vi "Andor_iXon_Init_Picture.vi"(8 "Input Cluster 2":T6) -> (0 "Output Cluster":T6)   [LabVIEW 2009]
uses:
  atmcd32d.llb/AcquisitionMode_mode typedef.ctl
  atmcd32d.llb/ReadMode_mode typedef.ctl
  atmcd32d.llb/TriggerMode_mode typedef.ctl
  atmcd32d.llb/Shutter_type typedef.ctl
  atmcd32d.llb/Shutter_mode typedef.ctl
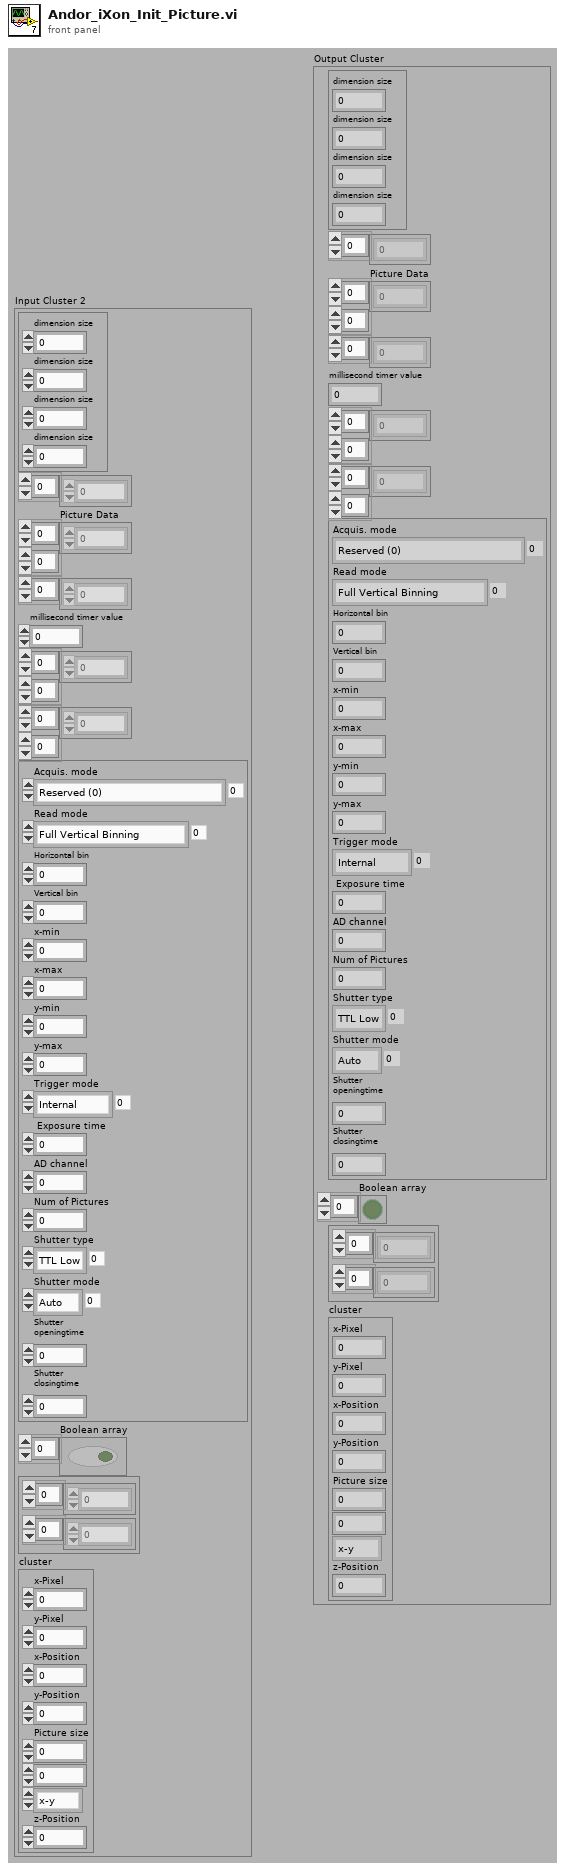
[diagram p1: front panel]
types:
  T1 = typedef "AcquisitionMode_mode typedef.ctl" = enum16{"Reserved (0)", "Single Scan", "Accumulate", "Kinetics", "Fast Kinetics", "Run Till Abort", "Reserved (6)", "Reserved (7)", "Reserved (8)", "Time Delayed Integration"}
  T2 = typedef "ReadMode_mode typedef.ctl" = enum16{"Full Vertical Binning", "Multi-Track", "Random-Track", "Single-Track", "Image"}
  T3 = typedef "TriggerMode_mode typedef.ctl" = enum16{"Internal", "External", "N/A (2)", "N/A (3)", "N/A (4)", "N/A (5)", "External Start"}
  T4 = typedef "Shutter_type typedef.ctl" = enum16{"TTL Low", "TTL High"}
  T5 = typedef "Shutter_mode typedef.ctl" = enum16{"Auto", "Open", "Close"}
  T6 = cluster{cluster{"dimension size":i32, "dimension size":i32, "dimension size":i32, "dimension size":i32}, i32[], "Picture Data":dbl[][], u32[], "millisecond timer value":u32, dbl[][], i32[][], cluster{"Acquis. mode":T1, "Read mode":T2, "Horizontal bin":i32, "Vertical bin":i32, "x-min":i32, "x-max":i32, "y-min":i32, "y-max":i32, "Trigger mode":T3, " Exposure time":sgl, "AD channel":i32, "Num of Pictures":i32, "Shutter type":T4, "Shutter mode":T5, "Shutter\nopeningtime":i32, "Shutter\nclosingtime":i32}, "Boolean array":bool[], cluster{dbl[], dbl[]}, "cluster":cluster{"x-Pixel":u16, "y-Pixel":u16, "x-Position":dbl, "y-Position":dbl, "Picture size":dbl, dbl, enum32{"x-y", "x-z", "y-z"}, "z-Position":dbl}}
  T7 = cluster{"Acquis. mode":T1, "Read mode":T2, "Horizontal bin":i32, "Vertical bin":i32, "x-min":i32, "x-max":i32, "y-min":i32, "y-max":i32, "Trigger mode":T3, " Exposure time":sgl, "AD channel":i32, "Num of Pictures":i32, "Shutter type":T4, "Shutter mode":T5, "Shutter\nopeningtime":i32, "Shutter\nclosingtime":i32}
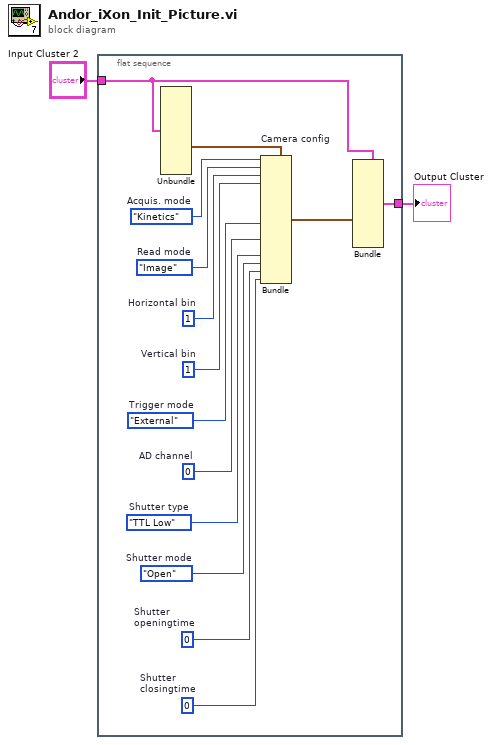
[diagram p0: block diagram]
diagram:
  n1 = flat-sequence {
    tunnel: "Input Cluster 2" -> [w4]
    tunnel: [w6] -> w2
    frame #0 {
      w10 = 1  # Vertical bin
      w9 = 1  # Horizontal bin
      w16 = 0  # Shutter closingtime
      w15 = 0  # Shutter openingtime
      w14 = Shutter_mode_typedef."Open"  # Shutter mode
      w13 = Shutter_type_typedef."TTL Low"  # Shutter type
      w12 = 0  # AD channel
      w11 = TriggerMode_mode_typedef."External"  # Trigger mode
      w8 = ReadMode_mode_typedef."Image"  # Read mode
      w7 = AcquisitionMode_mode_typedef."Kinetics"  # Acquis. mode
      n2 = Unbundle(w4) -> (w3:T7)  [unwired: 10 out]
      n3 = Bundle "Camera config"(cluster=w3, "Acquis. mode"=w7, "Read mode"=w8, "Horizontal bin"=w9, "Vertical bin"=w10, "Trigger mode"=w11, "AD channel"=w12, "Shutter type"=w13, "Shutter mode"=w14, "Shutter\nopeningtime"=w15, "Shutter\nclosingtime"=w16) -> (w5:T7)  [unwired: 6 out]
      n4 = Bundle(cluster=w4, w5) -> (w6:T6)  [unwired: 10 out]
    }
  }
  "Output Cluster" <- w2
